vi "IIR Filter for 1 Chan (CDB).vi"(4 "optional IIR filter specifications":T3={"Lower PB"=100.0, "Upper PB"=0.0, "Lower SB"=200.0, "Upper SB"=0.0, "PB Gain"=-3.0, "SB Gain"=-60.0, "Scale"=TRUE} {"PB Gain" format="%0.2f"; "SB Gain" format="%0.2f"; "Lower SB" format="%0.2p"; "Upper SB" format="%0.2f"; "Lower PB" format="%0.2p"; "Upper PB" format="%0.2f"}, 6 "IIR filter specifications":T4={"Topology"=enum."Butterworth", "Type"=enum."Lowpass", "Order"=1, "Lower Fc"=100.0, "Upper Fc"=200.0, "PB Ripple"=1.0, "SB Attenuation"=60.0} {"PB Ripple" format="%0.2f"; "SB Attenuation" format="%0.2f"; "Lower Fc" format="%0.2p"; "Upper Fc" format="%0.2p"}, 7 "reset filter":bool, 8 "error in (no error)":errorcluster, 10 "filter structure option":T1=10 items=["IIR 2nd Order"=0, "IIR 4th Order"=1, "Auto Select"=10], 11 "signal in":waveform(cdb)={"t0"=timestamp(0 s since 1904-01-01), "dt"=0.001, "Y"=[]}) -> (0 "error out":errorcluster, 2 "filter information":T2 {"phase H(w)"."df" format="%.2p"; "phase H(w)"."f0" format="%.2p"; "phase H(w)"."Phase H(w)" format="%.2p"; "magnitude H(w)"."df" format="%.2p"; "magnitude H(w)"."f0" format="%.2p"; "magnitude H(w)"."Mag H(w)" format="%.2p"}, 3 "signal out":waveform(cdb))   [LabVIEW 2020, in "NI_MAPro.lvlib"]
doc: "Filters signals in either single or multiple waveforms. If you are filtering multiple waveforms, the VI maintains separate filter states for each waveform. The data types you wire to the <B>signal in</B> and <B>IIR filter specifications</B> inputs determine the polymorphic instance to use."
uses:
  NI_MAPro.lvlib
  Filter Structure Type.ctl
  NI_MABase.lvlib
  NI_AALBase.lvlib
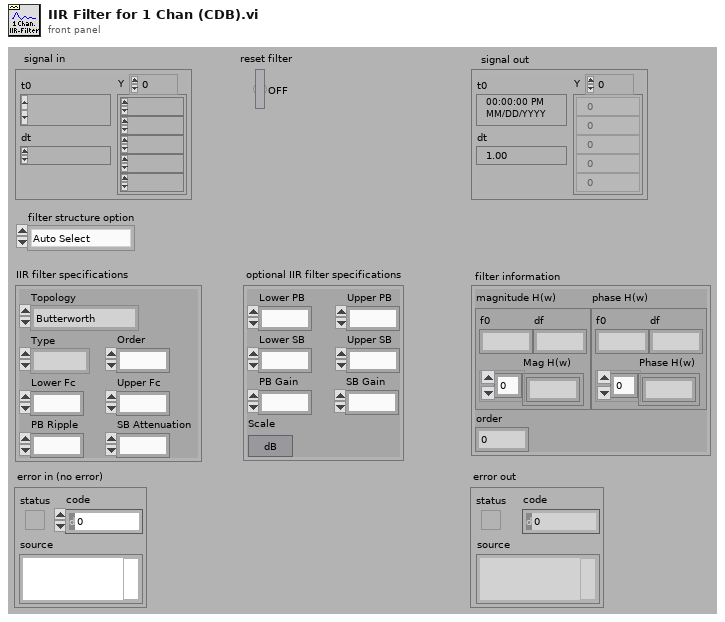
[diagram p1: front panel]
types:
  T1 = typedef "NI_AALBase.lvlib/Filter Structure Type.ctl" = u16
  T2 = cluster{"magnitude H(w)":cluster{"f0":dbl, "df":dbl, "Mag H(w)":dbl[]}, "phase H(w)":cluster{"f0":dbl, "df":dbl, "Phase H(w)":dbl[]}, "order":i32}
  T3 = cluster{"Lower PB":dbl, "Upper PB":dbl, "Lower SB":dbl, "Upper SB":dbl, "PB Gain":dbl, "SB Gain":dbl, "Scale":bool}
  T4 = cluster{"Topology":enum16{"Off", "Butterworth", "Chebyshev", "Inverse Chebyshev", "Elliptic", "Bessel"}, "Type":enum16{"Lowpass", "Highpass", "Bandpass", "Bandstop"}, "Order":i32, "Lower Fc":dbl, "Upper Fc":dbl, "PB Ripple":dbl, "SB Attenuation":dbl}
  T5 = cluster{"filter structure":enum32{"IIR 2nd Order", "IIR 4th Order"}, "Reverse Coefficients":dbl[], "Forward Coefficients":dbl[]}
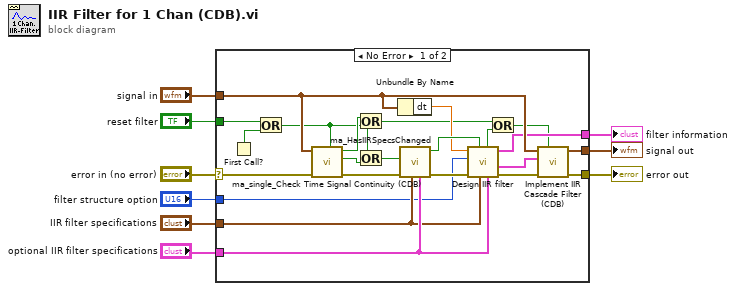
[diagram p0: block diagram]
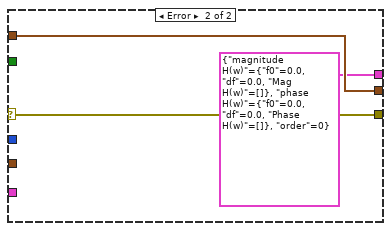
[diagram p2: hidden frame]
diagram:
  n1 = case shown="No Error" "error in (no error)" {
    selector: "error in (no error)" -> [w29 w34]
    tunnel: "signal in" -> [w31 w35]
    tunnel: [w32 w34] -> w8
    tunnel: [w30 w35] -> w7
    tunnel: [w28 T2 {"magnitude H(w)"={"f0"=0.0, "df"=0.0, "Mag H(w)"=[]}, "phase H(w)"={"f0"=0.0, "df"=0.0, "Phase H(w)"=[]}, "order"=0} ("Filter Information")] -> w5
    tunnel: "reset filter" -> [w13 _]
    tunnel: "optional IIR filter specifications" -> [w12 _]
    tunnel: "IIR filter specifications" -> [w11 _]
    tunnel: "filter structure option" -> [w10 _]
    frame No Error {
      n2 = First Call?() -> (First Call?: T/F=w15:bool)
      n3 = Or(x=w13, y=w15) -> (x .or. y?=w14:bool)
      n4 = call "ma_single_Check Time Signal Continuity (CDB).vi"("Ignore input time stamp"=w14, "error in (no error)"=w29, "Waveform"=w31) -> ("error out"=w23:errorcluster, "dt changed"=w18:bool, "t0 changed"=w17:bool)  [unwired: 5 in, 1 out]
      n5 = Or(x=w17, y=w14) -> (x .or. y?=w16:bool)
      n6 = Or(x=w14, y=w18) -> (x .or. y?=w19:bool)
      n7 = Unbundle By Name(w31) -> ("dt"=w20:dbl)
      n8 = call "ma_HasIIRSpecsChanged.vi"("optional IIR filter specifications"=w12, "IIR filter specifications"=w11, "error in (no error)"=w23, "redesign filter"=w19) -> ("error out"=w22:errorcluster, "ValsDifferent?"=w21:bool)  [unwired: 6 in]
      n9 = call "Design IIR filter.vi"("Optional IIR Filter Specifications"=w12, "IIR Filter specifications"=w11, "Redesign filter"=w21, "error in"=w22, "filter structure option"=w10, "dt"=w20) -> ("error out"=w27:errorcluster, "IIR Filter Cluster"=w26:T5, "Filter Information"=w28:T2, "Reset filter state"=w25:bool)  [unwired: 2 in]
      n10 = Or(x=w16, y=w25) -> (x .or. y?=w24:bool)
      n11 = call "Implement IIR Cascade Filter (CDB).vi"("Reset"=w24, "error in (no error)"=w27, "IIR Filter Cluster"=w26, "Waveform"=w31) -> ("error out"=w32:errorcluster, "Filtered Waveform"=w30:waveform(cdb))  [unwired: 6 in]
    }
    frame Error {
    }
  }
  "error out" <- w8
  "signal out" <- w7
  "filter information" <- w5
